vi "Error 5004.vi"(8 "error in (no error)":errorcluster, 10 "Proto file path":path) -> (0 "error out":errorcluster)   [LabVIEW 2020, in "gRPC Scripting Tools.lvlib"]
uses:
  gRPC Scripting Tools.lvlib
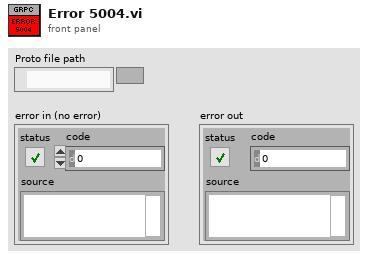
[diagram p1: front panel]
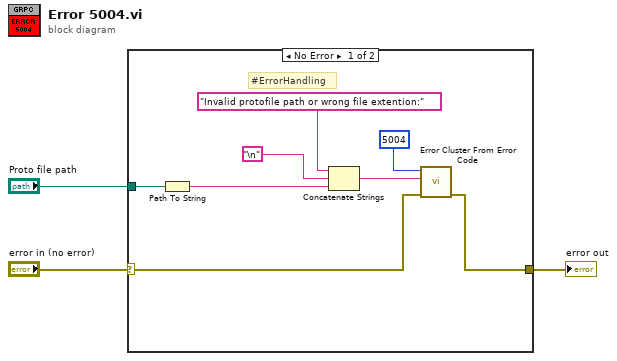
[diagram p0: block diagram]
diagram:
  n1 = case shown="No Error" "error in (no error)" {
    selector: "error in (no error)" -> [w4 w12]
    tunnel: [w11 w12] -> w3
    tunnel: "Proto file path" -> [w8 _]
    frame No Error {
      # "#ErrorHandling"
      n2 = Path To String(path=w8) -> (string=w9:string)
      n3 = Concatenate Strings("Invalid protofile path or wrong file extention:" ("error message (\"\")"), "\n", w9) -> (w10:string)
      n4 = call <vilib>:"Error Cluster From Error Code.vi"("error in (no error)"=w4, "error message (\"\")"=w10, "error code (0)"=5004) -> ("error out"=w11:errorcluster)  [unwired: 6 in]
    }
    frame Error {
    }
  }
  "error out" <- w3
